vi "REPORT_get_default_row_color.vi"(6 "row":i16) -> (3 "color":u32)   [LabVIEW 2019]
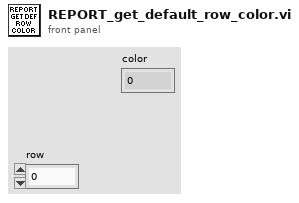
[diagram p1: front panel]
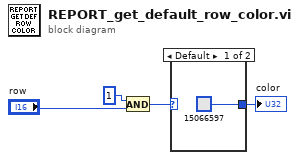
[diagram p0: block diagram]
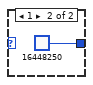
[diagram p2: hidden frame]
diagram:
  n1 = And(x=i16 1, y="row") -> (x .and. y?=w3:i16)
  n2 = case shown="Default" w3 {
    tunnel: [u32 15066597 u32 16448250] -> w1
    frame Default {
    }
    frame 1 {
    }
  }
  "color" <- w1
